vi "BASIC FPGA READ.vi"() -> ()   [LabVIEW 2016]
uses:
  Utilities/FPGA Interface/FPGA Interface.lvclass
panel:
  out "Data":u16[](array[numeric]) format="%04x"
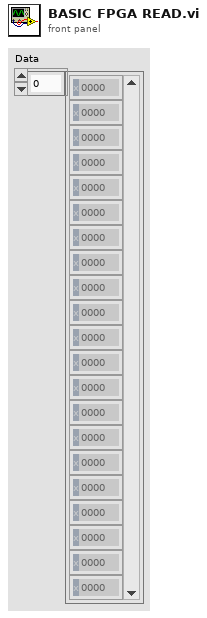
[diagram p1: front panel]
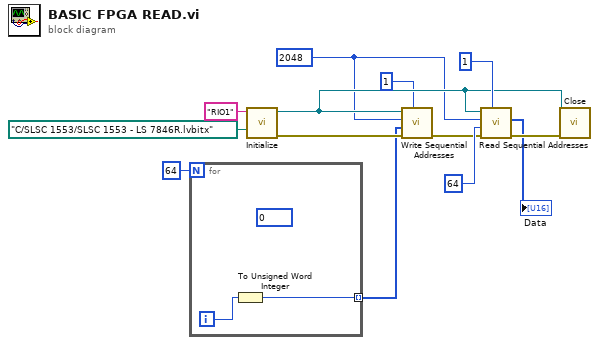
[diagram p0: block diagram]
diagram:
  w4 = u16 2048 ("Starting Address")
  n1 = for {
    N: 64 -> [_]
    tunnel: [w14] -> w2 mode=indexing
    i -> [w15]
    (unwired) u16 0 ("Starting Address")
    n2 = To Unsigned Word Integer(number=w15) -> (unsigned 16bit integer=w14:u16)
  }
  n3 = call "Initialize.vi"("Bitfile path"=path "C:/SLSC 1553/SLSC 1553 - LS 7846R.lvbitx", "Device address"="RIO1") -> ("error out"=w6:errorcluster, "FPGA Interface out"=w7:refnum<class "FPGA Interface.lvclass">)  [unwired: 8 in]
  n4 = call-dynamic "Write Sequential Addresses.vi"("Target IC (1-8)"=u8 1, "error in (no error)"=w6, "Data"=w2, "Starting Address"=w4, "FPGA Interface in"=w7) -> ("error out"=w5:errorcluster)  [unwired: 6 in]
  n5 = call-dynamic "Read Sequential Addresses.vi"("Target IC (1-8)"=u8 1, "error in (no error)"=w5, "Addresses to Read"=u16 64 ("Target IC (1-8)"), "Starting Address"=w4, "FPGA Interface in"=w7) -> ("error out"=w13:errorcluster, "Data"=→"Data":u16[])  [unwired: 5 in]
  n6 = call "Close.vi"("error in (no error)"=w13, "FPGA Interface in"=w7) -> ()  [unwired: 9 in, 1 out]
